vi "USBPT104Example.vi"() -> ()   [LabVIEW 2010]
panel:
  in  "Channel Filters":i16(ring) items=["Off", "On"]
  in  "SetMains":u16(ring) items=["50 Hz", "60 Hz"]
  out "Ch4 Status":enum32{"Red", "Yellow", "Green"}(radio)
  out "Ch3 Status":enum32{"Red", "Yellow", "Green"}(radio)
  out "GetValue PICO_STATUS log":T1(array[cluster]) {"Hex Code" format="%x"}
  out "Ch2 Status":enum32{"Red", "Yellow", "Green"}(radio)
  out "Ch1 Status":enum32{"Red", "Yellow", "Green"}(radio)
  out "CH4 Value":dbl(slide)=nan min=-200.0 max=800.0 scale=0.0..115.0
  out "CH3 Value":dbl(slide)=nan min=-200.0 max=800.0 scale=0.0..10000.0
  out "CH2 Value":dbl(slide)=nan min=-200.0 max=800.0 scale=0.0..10000.0
  out "CH1 Value":dbl(slide)=nan min=-200.0 max=800.0 scale=-200.0..800.0
  in  "Channel Settings":T2={"CH1 # Wires"=4, "CH1 Measurement Type"=1, "CH2 # Wires"=2, "CH2 Measurement Type"=0, "CH3 # Wires"=2, "CH3 Measurement Type"=0, "CH4 # Wires"=2, "CH4 Measurement Type"=0} {"CH4 Measurement Type" items=["OFF", "PT100", "PT1000", "Resistance to 375 Ohms", "Resistance to 10 kOhms", "Differential to 115 mV", "Differential to 2500 mV", "Single-ended to 115 mV", "Single-ended to 2500 mV"]; "CH4 # Wires" items=["2"=2, "3"=3, "4"=4]; "CH3 Measurement Type" items=["OFF", "PT100", "PT1000", "Resistance to 375 Ohms", "Resistance to 10 kOhms", "Differential to 115 mV", "Differential to 2500 mV", "Single-ended to 115 mV", "Single-ended to 2500 mV"]; "CH3 # Wires" items=["2"=2, "3"=3, "4"=4]; "CH2 Measurement Type" items=["OFF", "PT100", "PT1000", "Resistance to 375 Ohms", "Resistance to 10 kOhms", "Differential to 115 mV", "Differential to 2500 mV", "Single-ended to 115 mV", "Single-ended to 2500 mV"]; "CH2 # Wires" items=["2"=2, "3"=3, "4"=4]; "CH1 Measurement Type" items=["OFF", "PT100", "PT1000", "Resistance to 375 Ohms", "Resistance to 10 kOhms", "Differential to 115 mV", "Differential to 2500 mV", "Single-ended to 115 mV", "Single-ended to 2500 mV"]; "CH1 # Wires" items=["2"=2, "3"=3, "4"=4]}
  out "Unit Info":T3
  in  "Connection":bool=TRUE
  in  "Use Serial Number":bool
  in  "Serial Number":string
  in  "IP Address:port number":string="192.168.1.30:6250"
  out "PT-104 Units":string
  in  "error in (no error)":errorcluster
  out "End time":timestamp=timestamp(-9593251199.456087 s since 1904-01-01)
  out "Start time":timestamp=timestamp(-9593251199.456087 s since 1904-01-01)
  out "error out":errorcluster
  in  "Update settings":bool
  in  "Stop":bool
  # "USB"
  # "Ethernet"
  # "Channel Status LED-\nYellow- Waiting/Off\nGreen- Read OK\nRed- Read Error"
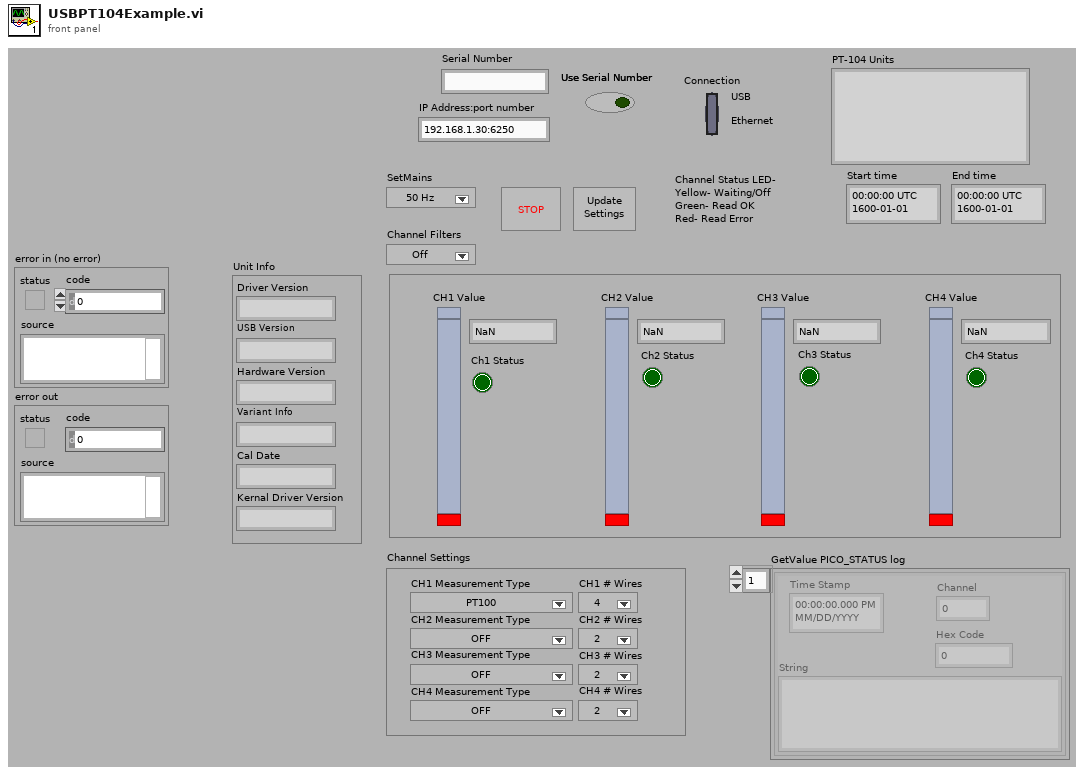
[diagram p1: front panel]
types:
  T1 = cluster{"Time Stamp":timestamp, "Hex Code":i32, "String":string, "Channel":i32}[]
  T2 = cluster{"CH1 # Wires":i16, "CH1 Measurement Type":i32, "CH2 # Wires":i16, "CH2 Measurement Type":i32, "CH3 # Wires":i16, "CH3 Measurement Type":i32, "CH4 # Wires":i16, "CH4 Measurement Type":i32}
  T3 = cluster{"Driver Version":string, "USB Version":string, "Hardware Version":string, "Variant Info":string, "Cal Date":string, "Kernal Driver Version":string, "NA":string, "NA 2":string, "NA":string, "NA 3":string, "NA 4":string, "NA 5":string, "NA 6":string, "NA 7":string, "NA 8":string}
  T4 = cluster{"seconds since 1Jan1904":timestamp, i32, "String":string, i32}[]
  T5 = cluster{"Channel Value":dbl, "Data Range:Maximum":dbl, "Scale.Range:Minimum":dbl}
  T6 = cluster{"seconds since 1Jan1904":timestamp, i32, "String":string, i32}
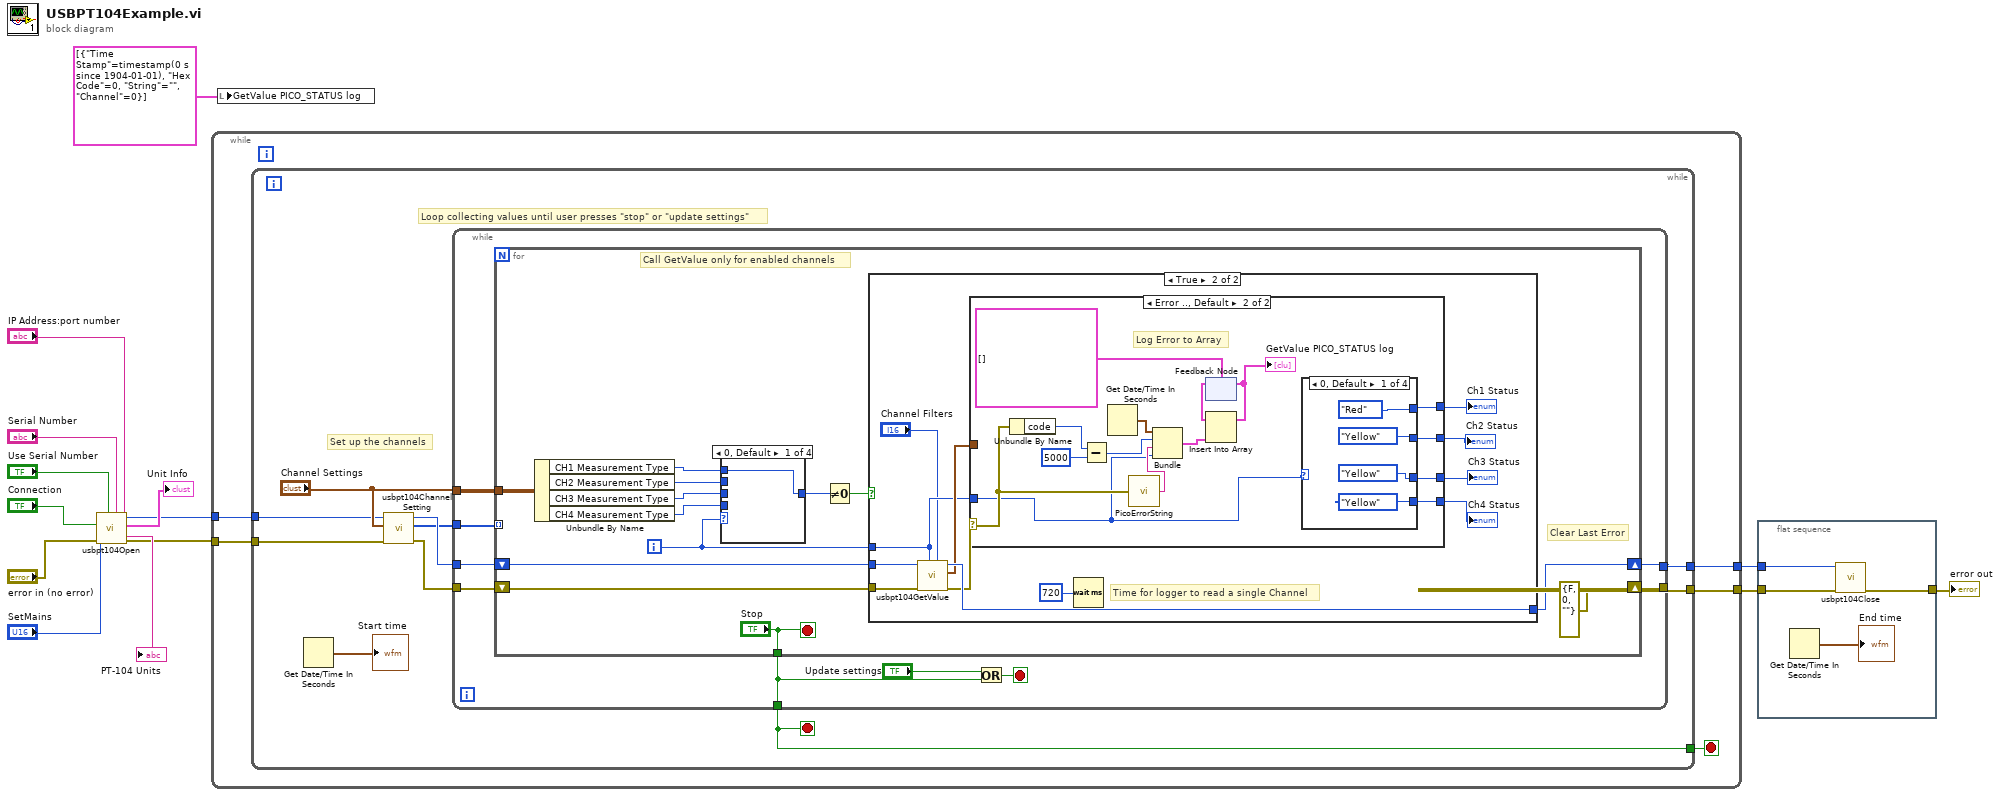
[diagram p0: block diagram]
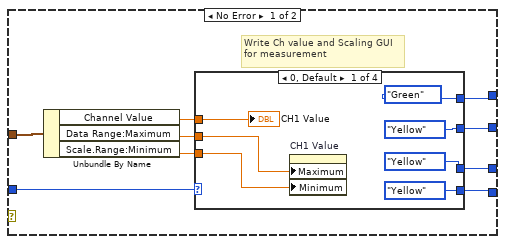
[diagram p6: hidden frame]
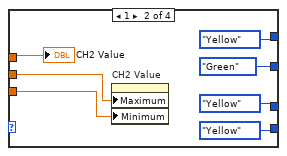
[diagram p7: hidden frame]
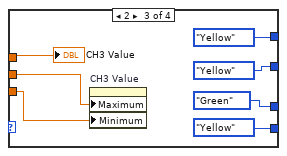
[diagram p8: hidden frame]
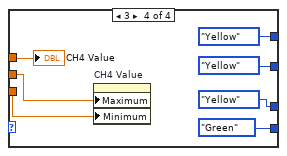
[diagram p9: hidden frame]
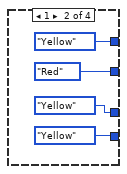
[diagram p10: hidden frame]
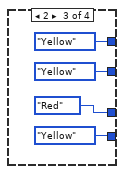
[diagram p11: hidden frame]
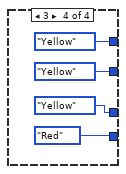
[diagram p12: hidden frame]
diagram:
  n1 = call "usbpt104Open.vi"("IP Address:port number"="IP Address:port number", "Serial Number"="Serial Number", "Use Serial Number"="Use Serial Number", "error in (no error)"="error in (no error)", "Connection"="Connection", "SetMains"="SetMains") -> ("error out"=w7:errorcluster, "Unit Info"=→"Unit Info":T3, "handle out"=w6:i16, "PT-104 Units"=→"PT-104 Units":string)  [unwired: 1 in, 1 out]
  n2 = while {
    tunnel: w7 -> [w19]
    tunnel: w6 -> [w18]
    tunnel: [w16] -> w5
    tunnel: [w15] -> w4
    stop <- w17 stop-if-true
    n3 = while {
      tunnel: [w29] -> w16
      tunnel: [w28] -> w15
      tunnel: [w24] -> w17
      tunnel: w19 -> [w23]
      tunnel: w18 -> [w22]
      stop <- w24 stop-if-true
      # "Loop collecting values until user presses \"stop\" or \"update settings\""
      # "Set up the channels"
      n4 = Get Date/Time In Seconds() -> (seconds since 1Jan1904=→"Start time":timestamp)
      n5 = call "usbpt104ChannelSetting.vi"("error in (no error)"=w23, "Channel Settings"="Channel Settings", "Handle In"=w22) -> ("error out"=w27:errorcluster, "Channel Enable Array"=w20:u8[], "Handle out"=w26:i16)  [unwired: 6 in]
      n6 = while {
        tunnel: w26 -> [w38]
        tunnel: w27 -> [w37]
        tunnel: [w34] -> w29
        tunnel: [w33] -> w28
        tunnel: [w31] -> w24
        tunnel: "Channel Settings" -> [w32]
        tunnel: w20 -> [w30]
        stop <- w36 stop-if-true
        n7 = for {
          shift-right: [errorcluster {"status"=FALSE, "code"=0, "source"=""} ("error out")] -> w34
          shift-left: w37 -> [w50]
          shift-right: [w47] -> w33
          shift-left: w38 -> [w51]
          tunnel: w32 -> [w45]
          tunnel: ["Stop"] -> w31
          tunnel: w30 -> [_] mode=indexing
          i -> [w46]
          stop <- "Stop" stop-if-true
          # "Clear Last Error"
          # "Call GetValue only for enabled channels"
          n8 = Unbundle By Name(w45) -> ("CH1 Measurement Type"=w44:i32, "CH2 Measurement Type"=w43:i32, "CH3 Measurement Type"=w42:i32, "CH4 Measurement Type"=w41:i32)
          n9 = case shown="0, Default" w46 {
            tunnel: [w52 w53 w54 w55] -> w48
            tunnel: w44 -> [w52 _ _ _]
            tunnel: w43 -> [_ w53 _ _]
            tunnel: w42 -> [_ _ w54 _]
            tunnel: w41 -> [_ _ _ w55]
            frame 0, Default {
            }
            frame 1 {
            }
            frame 2 {
            }
            frame 3 {
            }
          }
          n10 = Not Equal To 0?(x=w48) -> (x != 0?=w49:bool)
          n11 = case shown="True" w49 {
            tunnel: w51 -> [w56 w67]
            tunnel: w50 -> [_ w68]
            tunnel: [w56 w66] -> w47
            tunnel: w46 -> [_ w63]
            frame False {
            }
            frame True {
              # "Time for logger to read a single Channel"
              n12 = call "usbpt104GetValue.vi"("Filter"="Channel Filters", "Channel"=w63, "error in (no error)"=w68, "handle in"=w67) -> ("error out"=w62:errorcluster, "Channel Data"=w64:T5, "handle out"=w66:i16)  [unwired: 5 in]
              n13 = case shown="Error .., Default" w62 {
                selector: w62 -> [_ w112]
                tunnel: w64 -> [w77 _]
                tunnel: w63 -> [w76 w109]
                tunnel: [w72 w111] -> w61
                tunnel: [w71 w110] -> w60
                tunnel: [w69 w108] -> w59
                tunnel: [w70 w107] -> w58
                frame No Error {
                  # "Write Ch value and Scaling GUI for measurement"
                  n14 = Unbundle By Name(w77) -> ("Channel Value"=w75:dbl, "Data Range:Maximum"=w74:dbl, "Scale.Range:Minimum"=w73:dbl)
                  n15 = case shown="0, Default" w76 {
                    tunnel: w75 -> [w84 w91 w98 w105]
                    tunnel: w74 -> [w83 w90 w97 w104]
                    tunnel: w73 -> [w82 w89 w96 w103]
                    tunnel: [enum32{"Red", "Yellow", "Green"}."Green" ("Select") enum32{"Red", "Yellow", "Green"}."Yellow" ("Select") enum32{"Red", "Yellow", "Green"}."Yellow" ("Select") enum32{"Red", "Yellow", "Green"}."Yellow" ("Select")] -> w72
                    tunnel: [enum32{"Red", "Yellow", "Green"}."Yellow" ("Select") enum32{"Red", "Yellow", "Green"}."Green" ("Select") enum32{"Red", "Yellow", "Green"}."Yellow" ("Select") enum32{"Red", "Yellow", "Green"}."Yellow" ("Select")] -> w71
                    tunnel: [enum32{"Red", "Yellow", "Green"}."Yellow" ("Select") enum32{"Red", "Yellow", "Green"}."Yellow" ("Select") enum32{"Red", "Yellow", "Green"}."Yellow" ("Select") enum32{"Red", "Yellow", "Green"}."Green" ("Select")] -> w70
                    tunnel: [enum32{"Red", "Yellow", "Green"}."Yellow" ("Select") enum32{"Red", "Yellow", "Green"}."Yellow" ("Select") enum32{"Red", "Yellow", "Green"}."Green" ("Select") enum32{"Red", "Yellow", "Green"}."Yellow" ("Select")] -> w69
                    frame 0, Default {
                      n16 = property on="CH1 Value" class="Slide (strict)"("Maximum"=w83, "Minimum"=w82) -> ()  [unwired: 2 in, 2 out]
                      "CH1 Value" <- w84
                    }
                    frame 1 {
                      n17 = property on="CH2 Value" class="Slide (strict)"("Maximum"=w90, "Minimum"=w89) -> ()  [unwired: 2 in, 2 out]
                      "CH2 Value" <- w91
                    }
                    frame 2 {
                      n18 = property on="CH3 Value" class="Slide (strict)"("Maximum"=w97, "Minimum"=w96) -> ()  [unwired: 2 in, 2 out]
                      "CH3 Value" <- w98
                    }
                    frame 3 {
                      n19 = property on="CH4 Value" class="Slide (strict)"("Maximum"=w104, "Minimum"=w103) -> ()  [unwired: 2 in, 2 out]
                      "CH4 Value" <- w105
                    }
                  }
                }
                frame Error, Default {
                  # "Log Error to Array"
                  n20 = Unbundle By Name(w112) -> ("code"=w113:i32)
                  n21 = Subtract(x=w113, y=5000) -> (x-y=w115:i32)
                  n22 = Get Date/Time In Seconds() -> (seconds since 1Jan1904=w117:timestamp)
                  n23 = call "PicoErrorString.vi"("error in"=w112) -> ("String"=w116:string)  [unwired: 2 in, 2 out]
                  n24 = Bundle("seconds since 1Jan1904"=w117, w115, "String"=w116, w109) -> (w120:T6)  [unwired: 1 in]
                  n25 = feedback #1(T4 []) -> (w118:T4)
                  n26 = Insert Into Array(array=w118, new element=w120) -> (w119:T4)  [unwired: 1 in]
                  "GetValue PICO_STATUS log" <- w119
                  n27 = feedback-in #1(w119) -> ()
                  n28 = case shown="0, Default" w109 {
                    tunnel: [enum32{"Red", "Yellow", "Green"}."Red" ("Select") enum32{"Red", "Yellow", "Green"}."Yellow" ("Select") enum32{"Red", "Yellow", "Green"}."Yellow" ("Select") enum32{"Red", "Yellow", "Green"}."Yellow" ("Select")] -> w111
                    tunnel: [enum32{"Red", "Yellow", "Green"}."Yellow" ("Select") enum32{"Red", "Yellow", "Green"}."Red" ("Select") enum32{"Red", "Yellow", "Green"}."Yellow" ("Select") enum32{"Red", "Yellow", "Green"}."Yellow" ("Select")] -> w110
                    tunnel: [enum32{"Red", "Yellow", "Green"}."Yellow" ("Select") enum32{"Red", "Yellow", "Green"}."Yellow" ("Select") enum32{"Red", "Yellow", "Green"}."Red" ("Select") enum32{"Red", "Yellow", "Green"}."Yellow" ("Select")] -> w108
                    tunnel: [enum32{"Red", "Yellow", "Green"}."Yellow" ("Select") enum32{"Red", "Yellow", "Green"}."Yellow" ("Select") enum32{"Red", "Yellow", "Green"}."Yellow" ("Select") enum32{"Red", "Yellow", "Green"}."Red" ("Select")] -> w107
                    frame 0, Default {
                    }
                    frame 1 {
                    }
                    frame 2 {
                    }
                    frame 3 {
                    }
                  }
                }
              }
              "Ch1 Status" <- w61
              "Ch2 Status" <- w60
              "Ch3 Status" <- w59
              "Ch4 Status" <- w58
              n29 = Wait (ms)(milliseconds to wait=u32 720) -> ()  [unwired: 1 out]
            }
          }
        }
        n30 = Or(x="Update settings", y=w31) -> (x .or. y?=w36:bool)
      }
    }
  }
  n31 = local write "GetValue PICO_STATUS log"(T1 [{"Time Stamp"=timestamp(0 s since 1904-01-01), "Hex Code"=0, "String"="", "Channel"=0}] ("GetValue PICO_STATUS log")) -> ()
  n32 = flat-sequence {
    tunnel: w5 -> [w140]
    tunnel: [w138] -> w3
    tunnel: w4 -> [w139]
    frame #0 {
      n33 = Get Date/Time In Seconds() -> (seconds since 1Jan1904=→"End time":timestamp)
      n34 = call "usbpt104Close.vi"("error in (no error)"=w140, "handle in"=w139) -> ("error out"=w138:errorcluster)  [unwired: 8 in, 1 out]
    }
  }
  "error out" <- w3
